vi "dynanometer.vi"() -> ()   [LabVIEW 2013]
uses:
  <vilib>/Instr/_visa.llb/VISA Configure Serial Port (Instr).vi
panel:
  in  "VISA Port 2":refnum<visa-resource-name>
  in  "stop":bool
  in  "baud rate (9600)":u32=9600
  in  "VISA Port 1":refnum<visa-resource-name>
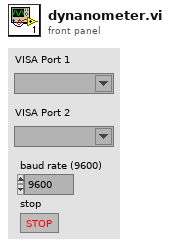
[diagram p1: front panel]
types:
  T1 = cluster{"pid":string, "data":cluster{"throttle":i32, "killswitch":i32}, "chksum":i32}
  T2 = cluster{"pid":string, "data":cluster{"engine":i32, "shaft":i32}, "chksum":i32}
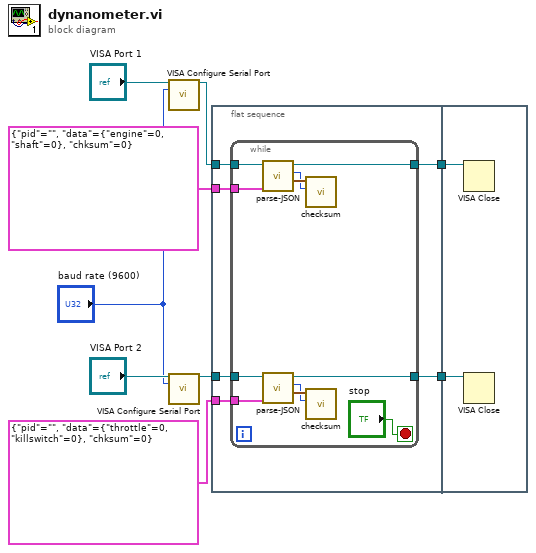
[diagram p0: block diagram]
diagram:
  n1 = call-poly "VISA Configure Serial Port"("VISA resource name"="VISA Port 1", "baud rate (9600)"="baud rate (9600)") -> ("VISA resource name out"=w8:refnum<visa-resource-name>)  [unwired: 12 in, 1 out]
  n2 = call-poly "VISA Configure Serial Port"("VISA resource name"="VISA Port 2", "baud rate (9600)"="baud rate (9600)") -> ("VISA resource name out"=w2:refnum<visa-resource-name>)  [unwired: 12 in, 1 out]
  n3 = flat-sequence {
    tunnel: w8 -> [w15]
    tunnel: [w14] -> w7
    tunnel: T2 {"pid"="", "data"={"engine"=0, "shaft"=0}, "chksum"=0} ("type and defaults") -> [w13]
    tunnel: T1 {"pid"="", "data"={"throttle"=0, "killswitch"=0}, "chksum"=0} ("type and defaults") -> [w12]
    tunnel: w2 -> [w11]
    tunnel: [w10] -> w1
    tunnel: w7 -> [w28]
    tunnel: w1 -> [w27]
    frame #0 {
      n4 = while {
        tunnel: w15 -> [w24]
        tunnel: [w26] -> w14
        tunnel: w13 -> [w23]
        tunnel: w12 -> [w20]
        tunnel: w11 -> [w22]
        tunnel: [w21] -> w10
        stop <- "stop" stop-if-true
        n5 = call "parse-JSON.vi"("JSON Structure (cluster)"=w23, "VISA resource name in"=w24) -> ("data"=w19:cluster{"engine":i32, "shaft":i32}, "chksum"=w18:i32, "VISA Refnum out"=w26:refnum<visa-resource-name>)  [unwired: 6 in, 1 out]
        n6 = call "parse-JSON.vi"("JSON Structure (cluster)"=w20, "VISA resource name in"=w22) -> ("data"=w17:cluster{"engine":i32, "shaft":i32}, "chksum"=w16:i32, "VISA Refnum out"=w21:refnum<visa-resource-name>)  [unwired: 6 in, 1 out]
        n7 = call "checksum.vi"("chksum"=w18, "data"=w19) -> ()  [unwired: 8 in, 2 out]
        n8 = call "checksum.vi"("chksum"=w16, "data"=w17) -> ()  [unwired: 8 in, 2 out]
      }
    }
    frame #1 {
      n9 = VISA Close(VISA resource name=w28) -> ()  [unwired: 1 in, 1 out]
      n10 = VISA Close(VISA resource name=w27) -> ()  [unwired: 1 in, 1 out]
    }
  }
